vi "Receipt.vi"(11 "read buffer":string) -> (2 "String":string, 3 "Boolean":bool)   [LabVIEW 2026]
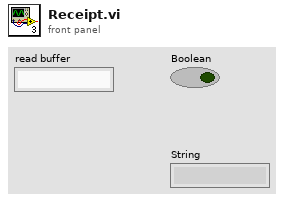
[diagram p1: front panel]
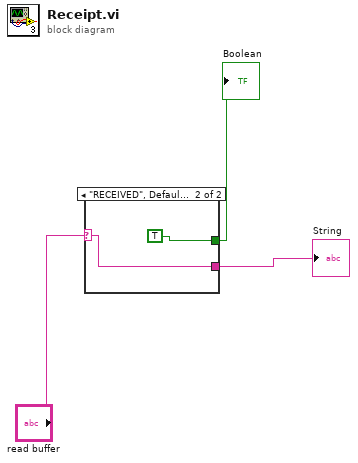
[diagram p0: block diagram]
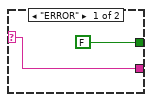
[diagram p2: hidden frame]
diagram:
  n1 = case shown="\"RECEIVED\", Default" "read buffer" {
    selector: "read buffer" -> [w5 w6]
    tunnel: [w5 w6] -> w3
    tunnel: [FALSE TRUE] -> w2
    frame "ERROR" {
    }
    frame "RECEIVED", Default {
    }
  }
  "String" <- w3
  "Boolean" <- w2
